vi "Initialize Attributes (public).vi"(8 "error in (no error)":errorcluster, 10 "Attribute Data":variant, 11 "CS++BaseActor in":refnum<class "CS++BaseActor.lvclass">) -> (0 "error out":errorcluster, 2 "Found?":bool, 3 "CS++BaseActor out":refnum<class "CS++BaseActor.lvclass">)   [LabVIEW 2015, in "CS++BaseActor.lvlib" / "CS++BaseActor.lvclass"]
doc: "Initialize object attribute.\n\nUnique resources should be allocated elsewhere!"
uses:
  CS++BaseActor.lvclass
  CS++BaseActor.lvclass/CS++BaseActor.ctl
  Libraries/Base/Severity.ctl
  Libraries/Base/CS++Base.lvlib
  Libraries/Utilities/CS++Utilities.lvlib
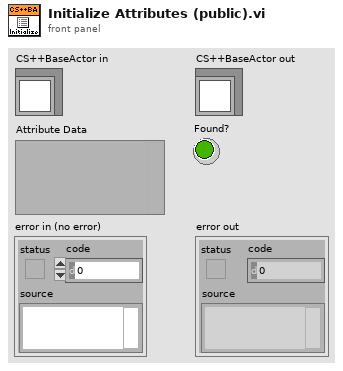
[diagram p1: front panel]
types:
  T1 = typedef "CS++Base.lvlib/Severity.ctl" = enum16{"emergency", "alert", "critical", "error", "warning", "notice", "info", "debug"}
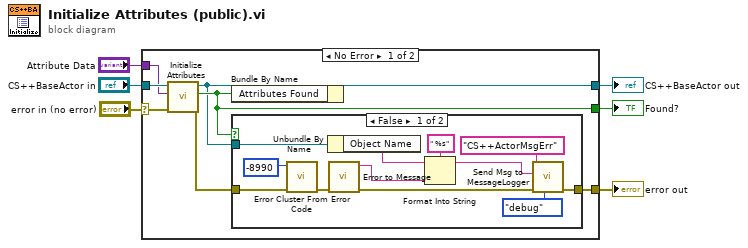
[diagram p0: block diagram]
diagram:
  n1 = case shown="No Error" "error in (no error)" {
    selector: "error in (no error)" -> [w14 w29]
    tunnel: [w7 w29] -> w5
    tunnel: [w11 w28] -> w3
    tunnel: "CS++BaseActor in" -> [w13 w28]
    tunnel: "Attribute Data" -> [w12 _]
    tunnel: [w10 _] -> w1
    frame No Error {
      n2 = call-dynamic "Initialize Attributes.vi"("error in (no error)"=w14, "Attribute Data"=w12, "CS++BaseActor in"=w13) -> ("error out"=w8:errorcluster, "Found?"=w10:bool, "CS++BaseActor out"=w9:refnum<class "CS++BaseActor.lvclass">)  [unwired: 6 in]
      n3 = Bundle By Name(cluster=w9, "Attributes Found"=w10) -> (w11:refnum<class "CS++BaseActor.lvclass">)
      n4 = case shown="False" w10 {
        tunnel: w8 -> [w18 w27]
        tunnel: w9 -> [w25 _]
        tunnel: [w15 w27] -> w7
        frame False {
          n5 = call <vilib>:"Error Cluster From Error Code.vi"("error in (no error)"=w18, "error code (0)"=-8990 ("Error Code (0)")) -> ("error out"=w17:errorcluster)  [unwired: 7 in]
          n6 = Unbundle By Name(w25) -> ("Object Name"=w22:string)
          n7 = call "Error to Message.vi"("Error In"=w17) -> ("Error Out"=w24:errorcluster, "Error Message"=w21:string)  [unwired: 9 in]
          n8 = Format Into String(format string=" %s", initial string=w22, w21) -> (resulting string=w19:string)  [unwired: 1 in, 1 out]
          n9 = call "Send Msg to MessageLogger.vi"("Severity Code (info)"=Severity."debug", "Error In"=w24, "Message Content"=w19, "Message Tag"="CS++ActorMsgErr") -> ("Error Out"=w15:errorcluster)  [unwired: 7 in]
        }
        frame True {
        }
      }
    }
    frame Error {
    }
  }
  "error out" <- w5
  "CS++BaseActor out" <- w3
  "Found?" <- w1
